vi "Filter for Enum Controls.vi"(8 "error in":errorcluster, 11 "controls":refnum<vi>[](array[refnum])) -> (0 "error out":errorcluster, 3 "enum controls and labels":T1(array[cluster]))   [LabVIEW 2020, in "Plug-In SDK Measurement.lvlib"]
uses:
  Plug-In SDK Measurement.lvlib
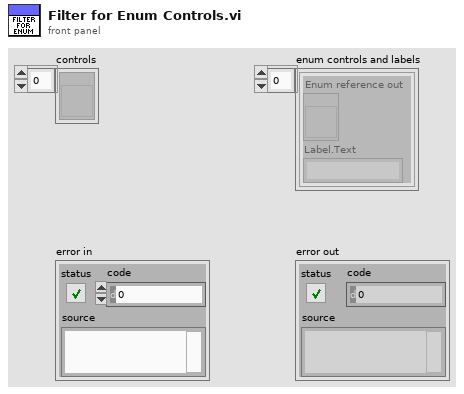
[diagram p1: front panel]
types:
  T1 = cluster{"Enum reference out":refnum<vi>, "Label.Text":string}[]
  T2 = cluster{"Enum reference out":refnum<vi>, "Label.Text":string}
  T3 = cluster{"enum reference out":refnum<vi>, "Label.Text":string}
  T4 = cluster{"enum reference out":refnum<vi>, "Label.Text":string}[]
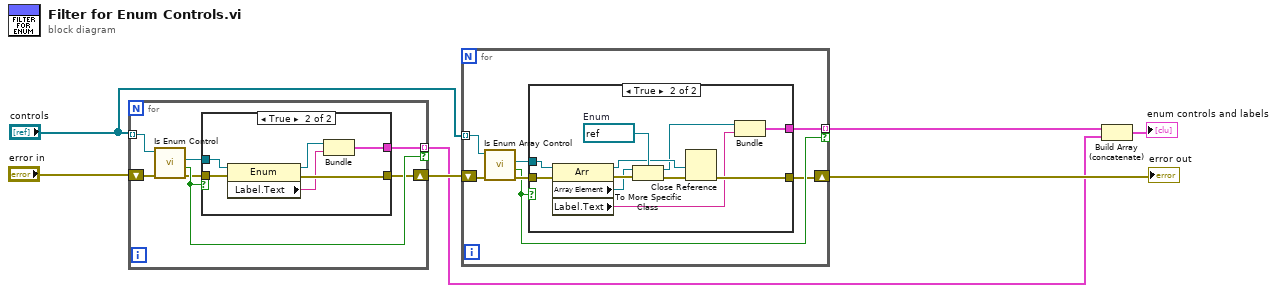
[diagram p0: block diagram]
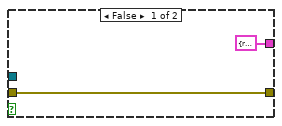
[diagram p2: hidden frame]
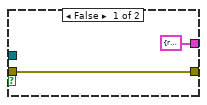
[diagram p3: hidden frame]
diagram:
  n1 = for {
    tunnel: "controls" -> [w13] mode=indexing
    tunnel: [w8] -> w2 mode=indexing if=w12
    shift-right: [w11] -> w6
    shift-left: "error in" -> [w14]
    n2 = call "Is Enum Control.vi"("error in"=w14, "control reference in"=w13) -> ("error out"=w10:errorcluster, "is enum control"=w12:bool, "enum reference out"=w9:refnum<vi>)  [unwired: 6 in, 1 out]
    n3 = case shown="True" w12 {
      tunnel: [w16 w21] -> w11
      tunnel: w10 -> [w16 w22]
      tunnel: w9 -> [_ w20]
      tunnel: [T2 {"Enum reference out"=refnum, "Label.Text"=""} w17] -> w8
      frame False {
      }
      frame True {
        n4 = property class="Enum"(reference=w20, error in=w22) -> (reference out=w19:refnum<vi>, error out=w21:errorcluster, "Label.Text"=w18:string)
        n5 = Bundle("enum reference out"=w19, "Label.Text"=w18) -> (w17:T3)  [unwired: 1 in]
      }
    }
  }
  n6 = for {
    tunnel: "controls" -> [w28] mode=indexing
    shift-right: [w25] -> w4
    shift-left: w6 -> [w29]
    tunnel: [w23] -> w3 mode=indexing if=w26
    n7 = call "Is Enum Array Control.vi"("error in)"=w29, "control reference in"=w28) -> ("error out"=w27:errorcluster, "is enum array control"=w26:bool, "array reference out"=w24:refnum<vi>)  [unwired: 6 in, 1 out]
    n8 = case shown="True" w26 {
      tunnel: w27 -> [w31 w41]
      tunnel: [w31 w35] -> w25
      tunnel: w24 -> [_ w38]
      tunnel: [cluster{refnum<vi>, "Label.Text":string} {refnum, "Label.Text"=""} w32] -> w23
      frame False {
      }
      frame True {
        w42 = refnum<vi> refnum  # Enum
        n9 = property class="Arr"(reference=w38, error in=w41) -> (reference out=w37:refnum<vi>, error out=w40:errorcluster, "Array Element"=w39:refnum<vi>, "Label.Text"=w34:string)
        n10 = To More Specific Class(target class=w42, reference=w39, error in=w40) -> (specific class reference=w33:refnum<vi>, error out=w36:errorcluster)
        n11 = Close Reference(reference=w37, error in (no error)=w36) -> (error out=w35:errorcluster)
        n12 = Bundle(w33, "Label.Text"=w34) -> (w32:cluster{refnum<vi>, "Label.Text":string})  [unwired: 1 in]
      }
    }
  }
  "error out" <- w4
  n13 = Build Array (concatenate)(w3, w2) -> (→"enum controls and labels":T4)
